vi "LEP_RV_OnStop.vi"() -> ()   [LabVIEW 2011]
doc: "Download and execute built VxWorks downloadable module and attach the LabVIEW Embedded debuger."
panel:
  out "error out":errorcluster
  in  "error in (no error)":errorcluster
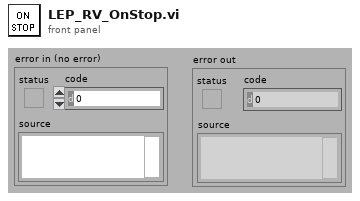
[diagram p1: front panel]
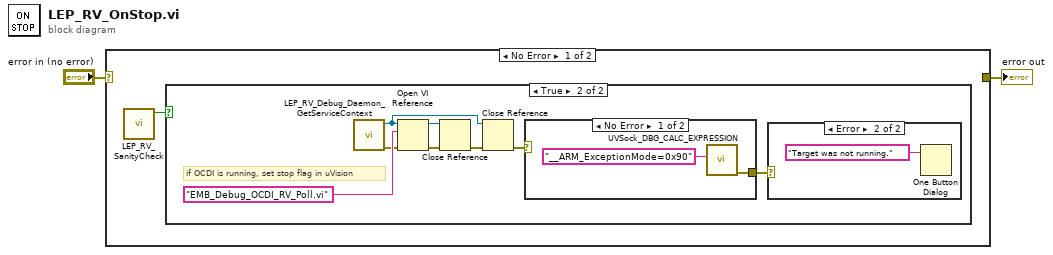
[diagram p0: block diagram]
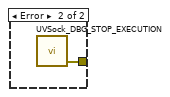
[diagram p3: hidden frame]
diagram:
  n1 = case shown="No Error" "error in (no error)" {
    selector: "error in (no error)" -> [_ w16]
    tunnel: [_ w16] -> w2
    frame No Error {
      n2 = call "LEP_RV_SanityCheck.vi"() -> ("ok"=w3:bool)  [unwired: 10 in, 1 out]
      n3 = case shown="True" w3 {
        frame False {
        }
        frame True {
          # "if OCDI is running, set stop flag in uVision"
          n4 = call "LEP_RV_Debug_Daemon_GetServiceContext.vi"() -> ("error out"=w7:errorcluster, "service context"=w4:refnum<vi>)  [unwired: 1 in, 9 out]
          n5 = Open VI Reference(application reference (local)=w4, vi path="EMB_Debug_OCDI_RV_Poll.vi", error in (no error)=w7) -> (vi reference=w9:refnum<vi>, error out=w8:errorcluster)  [unwired: 3 out]
          n6 = Close Reference(reference=w9, error in (no error)=w8) -> (error out=w6:errorcluster)
          n7 = Close Reference(reference=w4, error in (no error)=w6) -> (error out=w5:errorcluster)
          n8 = case shown="No Error" w5 {
            tunnel: [w12 w14] -> w11
            frame No Error {
              n9 = call "UVSock_DBG_CALC_EXPRESSION.vi"("Expression"="__ARM_ExceptionMode=0x90") -> ("error out"=w12:errorcluster)  [unwired: 2 in, 8 out]
            }
            frame Error {
              n10 = call "UVSock_DBG_STOP_EXECUTION.vi"() -> ("error out"=w14:errorcluster)  [unwired: 2 in, 3 out]
            }
          }
          n11 = case shown="Error" w11 {
            frame No Error {
            }
            frame Error {
              n12 = One Button Dialog(message="Target was not running.") -> ()  [unwired: 2 out]
            }
          }
        }
      }
    }
    frame Error {
    }
  }
  "error out" <- w2
